vi "SVT Initialize Swept Sine Task (DAQmx).vi"   [LabVIEW 2017, in "SoundVib_SweptSine.lvlib"]
doc: "Initializes swept-sine-analysis parameters on analog input and output devices."
uses:
  <vilib>/addons/Sound and Vibration/svt_Swept Sine/SoundVib_SweptSine.lvlib
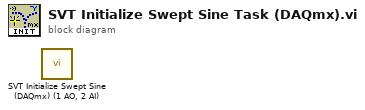
[diagram p0: block diagram]
diagram:
  n1 = call <vilib>:"SVT Initialize Swept Sine (DAQmx) (1 AO, 2 AI).vi"() -> ()  [unwired: 10 in, 2 out]
